vi "HW_GEN - Insert Data to Queue.vi"(8 "error in":errorcluster, 10 "data":T1, 11 "Object Name":string) -> (0 "error out":errorcluster, 3 "Object Name":string)   [LabVIEW 2016]
uses:
  Ctrls/HardWare _ Queue Data Type.ctl
panel:
  # "Data Out"
  # "Data In"
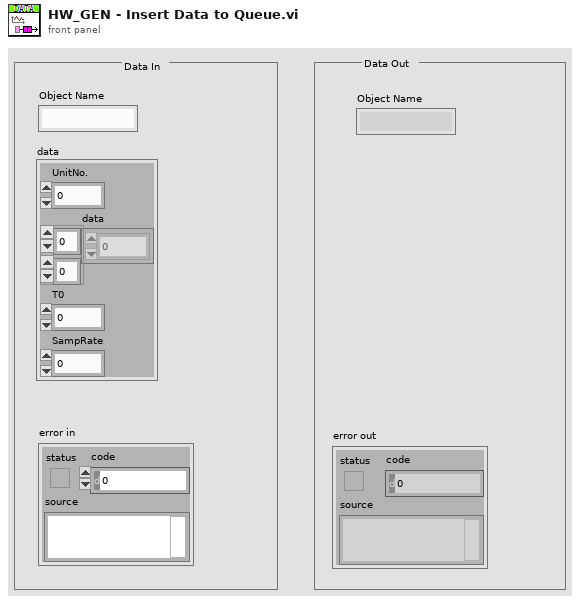
[diagram p1: front panel]
types:
  T1 = typedef "HardWare _ Queue Data Type.ctl" = cluster{"UnitNo.":i32, "data":dbl[][], "T0":dbl, "SampRate":dbl}
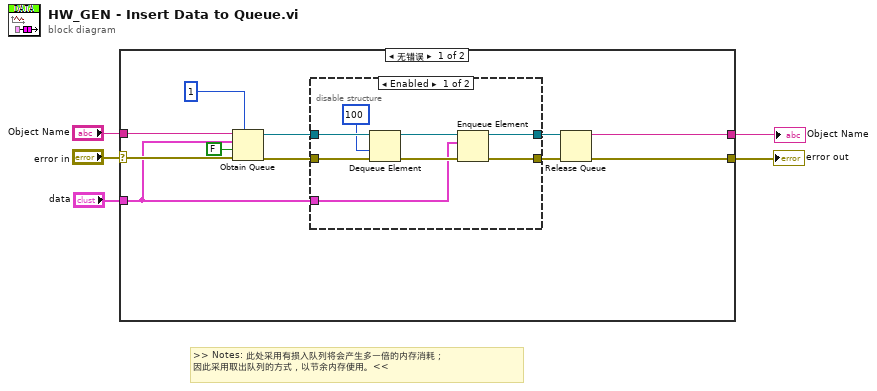
[diagram p0: block diagram]
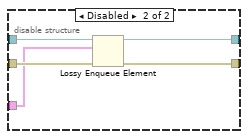
[diagram p2: hidden frame]
diagram:
  # ">> Notes: 此处采用有损入队列将会产生多一倍的内存消耗；\n因此采用取出队列的方式，以节余内存使用。<<"
  n1 = case shown="无错误" "error in" {
    selector: "error in" -> [w14 w31]
    tunnel: [w6 w31] -> w5
    tunnel: "Object Name" -> [w11 w30]
    tunnel: "data" -> [w7 _]
    tunnel: [w8 w30] -> w2
    frame No Error {
      n2 = Obtain Queue(max queue size (-1, unlimited)=1 ("队列最大值（-1，无限）"), name (unnamed)=w11, element data type=w7, create if not found? (T)=FALSE ("如未找到是否创建？(T)"), error in (no error)=w14) -> (queue out=w16:refnum<queue>, error out=w13:errorcluster)  [unwired: 1 out]
      n3 = disable-structure shown="Enabled" {
        disable-tunnel: w16 -> [w24 w29]
        disable-tunnel: w13 -> [w22 w28]
        disable-tunnel: [w20 w27] -> w10
        disable-tunnel: [w19 w26] -> w9
        disable-tunnel: w7 -> [w18 w25]
        frame Enabled {
          n4 = Dequeue Element(queue=w24, timeout in ms (-1)=100 ("超时毫秒(-1)"), error in (no error)=w22) -> (queue out=w23:refnum<queue>, error out=w21:errorcluster)  [unwired: 2 out]
          n5 = Enqueue Element(queue=w23, element=w18, error in (no error)=w21) -> (queue out=w19:refnum<queue>, error out=w20:errorcluster)  [unwired: 1 in, 1 out]
        }
        frame Disabled {
          n6 = Lossy Enqueue Element(queue=w29, element=w25, error in (no error)=w28) -> (queue out=w26:refnum<queue>, error out=w27:errorcluster)  [unwired: 2 out]
        }
      }
      n7 = Release Queue(queue=w9, error in (no error)=w10) -> (queue name=w8:string, error out=w6:errorcluster)  [unwired: 1 in, 1 out]
    }
    frame Error {
    }
  }
  "error out" <- w5
  "Object Name" <- w2
